vi "(SubVI) merge deep text.vi"(1 "Cluster":T1) -> (0 "merge text":string)   [LabVIEW 2022 SP3]
uses:
  <vilib>/Utility/error.llb/Trim Whitespace One-Sided.vi
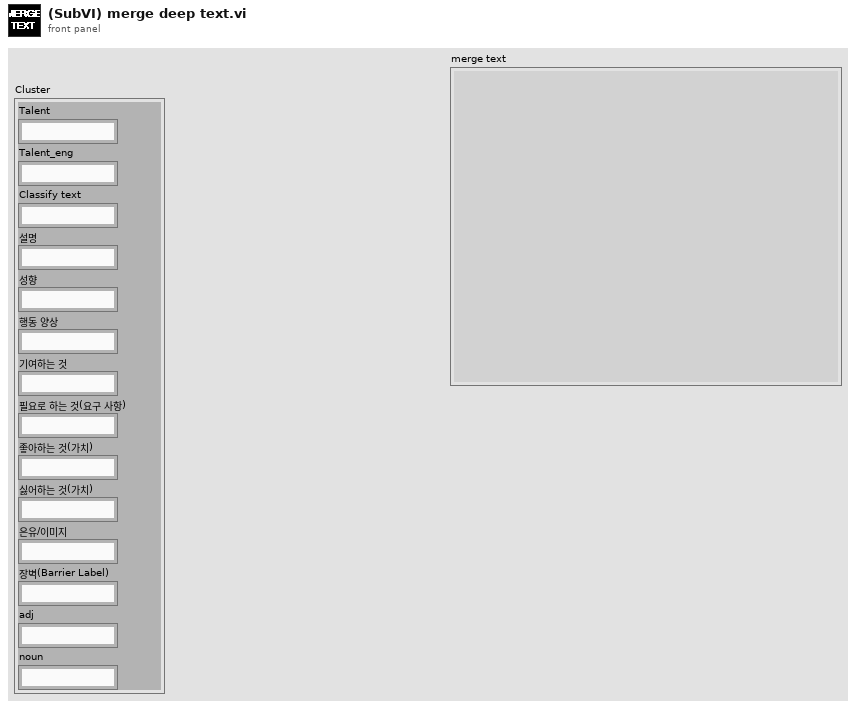
[diagram p1: front panel]
types:
  T1 = cluster{"Talent":string, "Talent_eng":string, "Classify text":string, "설명":string, "성향":string, "행동 양상":string, "기여하는 것":string, "필요로 하는 것(요구 사항)":string, "좋아하는 것(가치)":string, "싫어하는 것(가치)":string, "은유/이미지":string, "장벽(Barrier Label)":string, "adj":string, "noun":string}
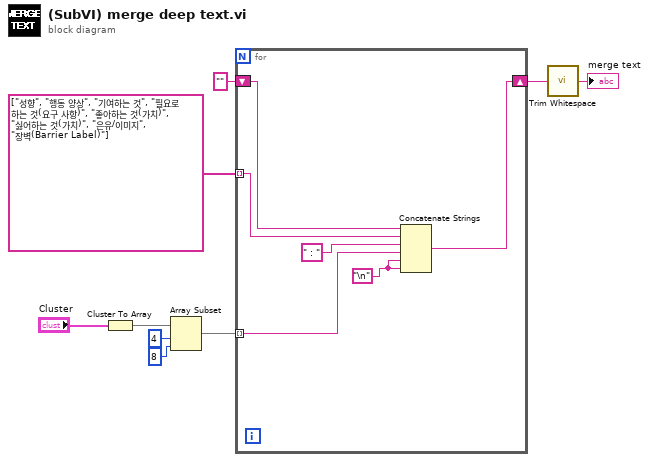
[diagram p0: block diagram]
diagram:
  n1 = Cluster To Array(cluster="Cluster") -> (array=w9:string[])
  n2 = Array Subset(array=w9, index=4, length=8) -> (w3:string[])
  n3 = for {
    tunnel: string[] ["성향", "행동 양상", "기여하는 것", "필요로 하는 것(요구 사항)", "좋아하는 것(가치)", "싫어하는 것(가치)", "은유/이미지", "장벽(Barrier Label)"] ("subarray") -> [w15] mode=indexing
    shift-right: [w12] -> w2
    shift-left: "" -> [w13]
    tunnel: w3 -> [w11] mode=indexing
    w10 = "\n"
    n4 = Concatenate Strings(w13, w15, " : ", w11, w10, w10) -> (w12:string)
  }
  n5 = call <vilib>:"Trim Whitespace.vi"("string"=w2) -> ("trimmed string"=→"merge text":string)  [unwired: 1 in]
